vi "reset_cRIO.vi"() -> ()   [LabVIEW 2015]
panel:
  out "Boolean 2":bool
  out "s? t:f":i32
  in  "Boolean":bool
  in  "stop":bool
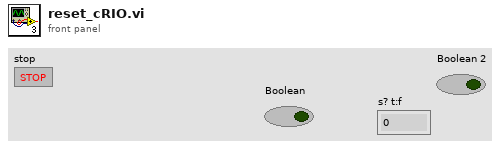
[diagram p1: front panel]
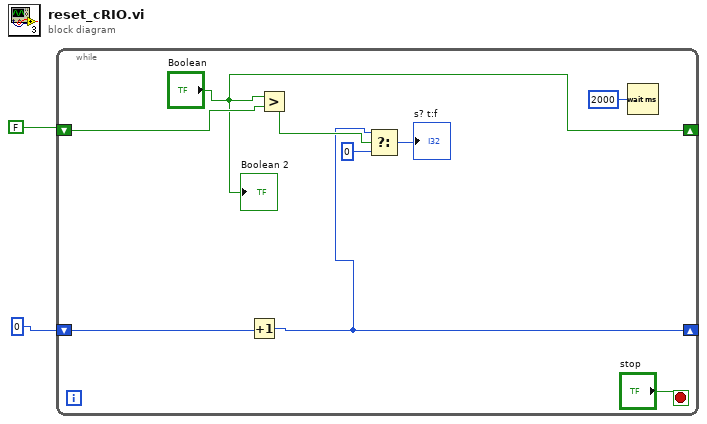
[diagram p0: block diagram]
diagram:
  n1 = while {
    shift-right: [w4] -> _
    shift-left: 0 -> [w10]
    shift-right: ["Boolean"] -> _
    shift-left: FALSE -> [w8]
    stop <- "stop" stop-if-true
    n2 = Increment(x=w10) -> (x+1=w4:i32)
    n3 = Greater?(x="Boolean", y=w8) -> (0:w7:bool)
    n4 = Select(t=w4, s=w7, f=0) -> (s? t:f=→"s? t:f":i32)
    n5 = Wait (ms)(milliseconds to wait=u32 2000) -> ()  [unwired: 1 out]
    "Boolean 2" <- "Boolean"
  }
